vi "CheckForDLL.vi"(8 "error in":errorcluster) -> (0 "error out":errorcluster)   [LabVIEW 2019, in "MicronGRPCClient.lvclass"]
uses:
  MicronGRPCClient.lvclass
  <vilib>/gRPC/LabVIEW gRPC Library/grpc-lvsupport-release.lvlib
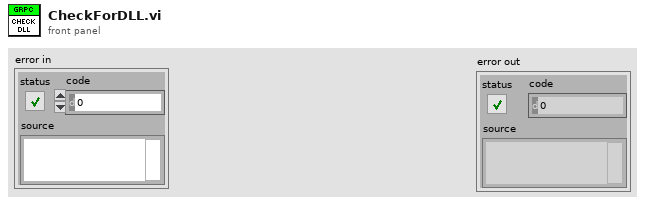
[diagram p1: front panel]
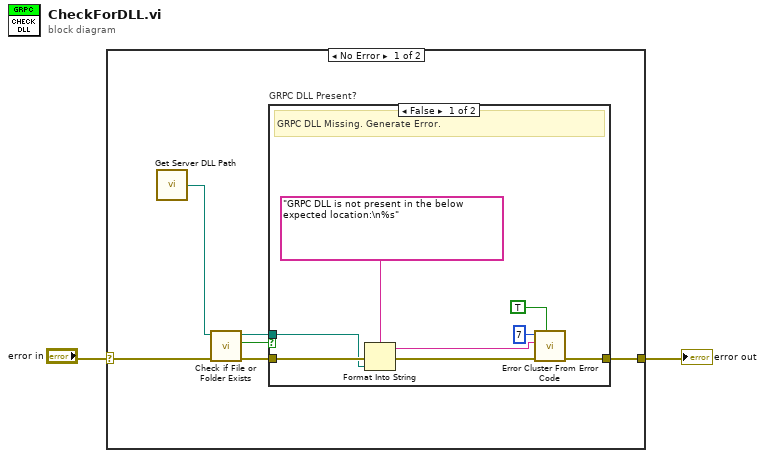
[diagram p0: block diagram]
diagram:
  n1 = case shown="No Error" "error in" {
    selector: "error in" -> [w8 w18]
    tunnel: [w5 w18] -> w1
    frame No Error {
      n2 = call <vilib>:"Get Server DLL Path.vi"() -> ("server dll path"=w7:path)
      n3 = call <vilib>:"Check if File or Folder Exists.vi"("error in (no error)"=w8, "path"=w7) -> ("error out"=w6:errorcluster, "file or folder exists?"=w4:bool, "dup path"=w3:path)  [unwired: 7 in]
      n4 = case "GRPC DLL Present?" shown="False" w4 {
        tunnel: w6 -> [w16 w17]
        tunnel: [w15 w17] -> w5
        tunnel: w3 -> [w11 _]
        frame False {
          # "GRPC DLL Missing. Generate Error."
          n5 = Format Into String(format string="GRPC DLL is not present in the below expected location:\n%s", error in=w16, w11) -> (resulting string=w10:string, error out=w12:errorcluster)  [unwired: 1 in]
          n6 = call <vilib>:"Error Cluster From Error Code.vi"("show call chain? (False)"=TRUE, "error in (no error)"=w12, "error message (\"\")"=w10, "error code (0)"=7) -> ("error out"=w15:errorcluster)  [unwired: 5 in]
        }
        frame True {
        }
      }
    }
    frame Error {
    }
  }
  "error out" <- w1
